vi "Run.vi"(8 "error in (no error)":errorcluster caption="entrée d'erreur (pas d'erreur)", 9 "Y":string[][](array[string]), 10 "X":string[][](array[string]), 11 "Argmin.lvclass":refnum<class "Argmin.lvclass">) -> (0 "error out":errorcluster caption="sortie d'erreur", 2 "Data":T1, 3 "Argmin.lvclass":refnum<class "Argmin.lvclass">)   [LabVIEW 2020, in "Argmin.lvclass"]
doc: "Returns : \n\n- argmin : numpy.ndarray\nY[argmin[i], :] is the row in Y that is closest to X[i, :]."
uses:
  Argmin.lvclass
  Argmin.lvclass/Argmin.ctl
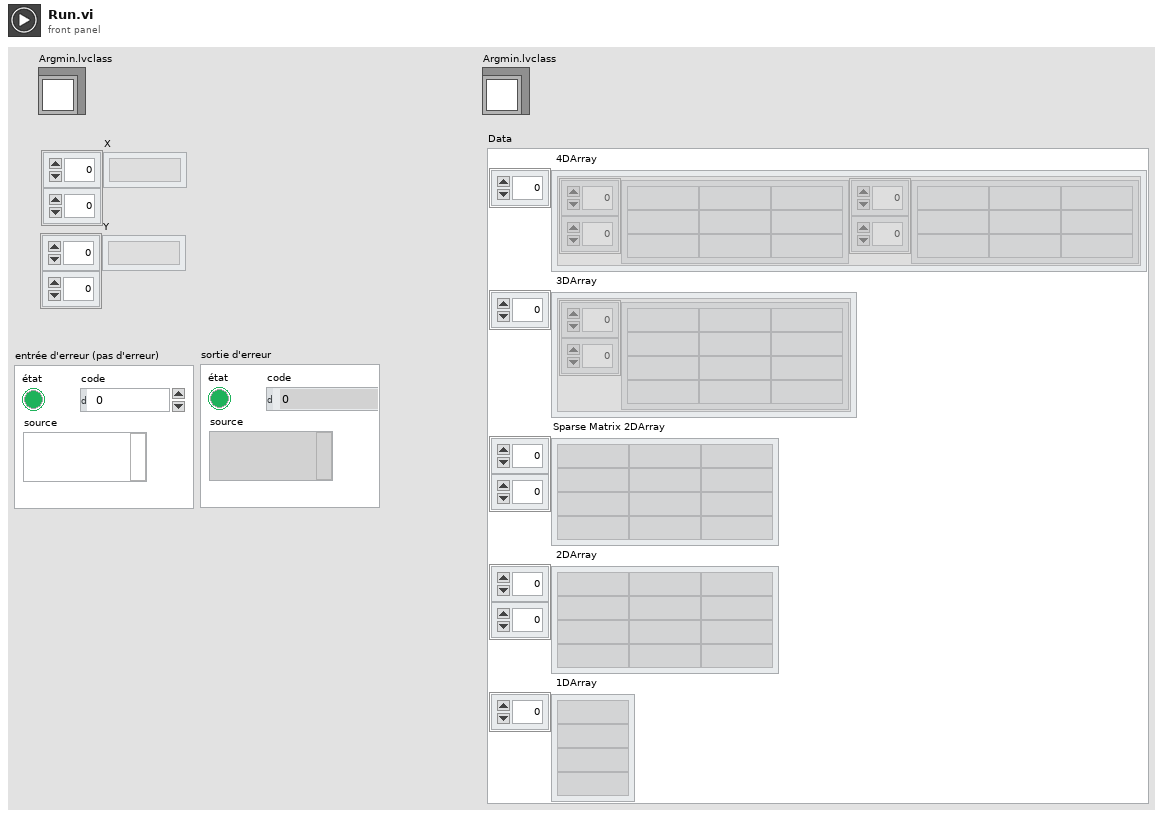
[diagram p1: front panel]
types:
  T1 = cluster{" 4DArray":cluster{"1":string[][], "2":string[][]}[], " 3DArray":cluster{"Tableau":string[][]}[], "Sparse Matrix 2DArray":string[][], " 2DArray":string[][], " 1DArray":string[]}
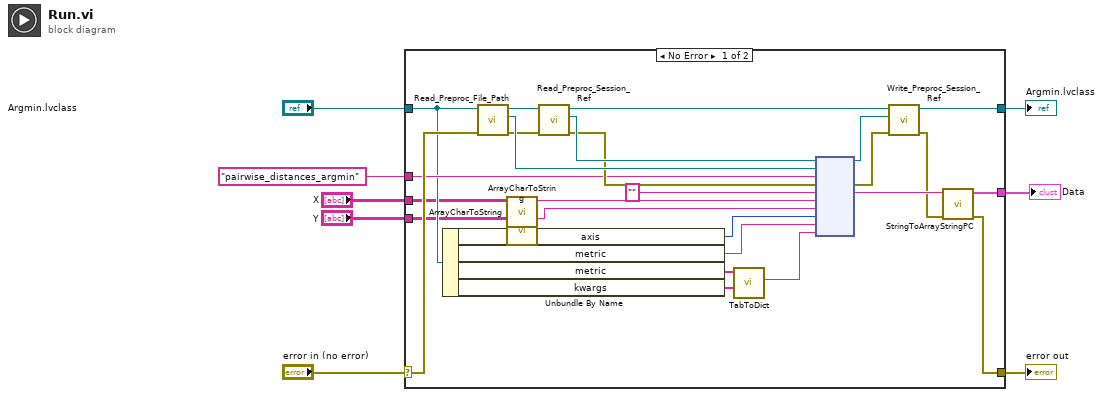
[diagram p0: block diagram]
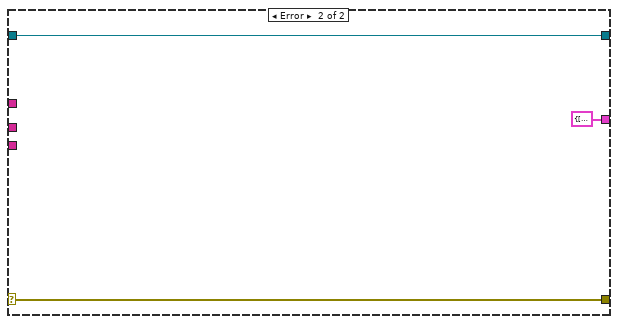
[diagram p2: hidden frame]
diagram:
  n1 = case shown="No Error" "error in (no error)" {
    selector: "error in (no error)" -> [w25 w37]
    tunnel: [w10 w37] -> w7
    tunnel: [w13 w36] -> w5
    tunnel: "Argmin.lvclass" -> [w23 w36]
    tunnel: "pairwise_distances_argmin" ("Fonction") -> [w24 _]
    tunnel: "X" -> [w17 _]
    tunnel: "Y" -> [w16 _]
    tunnel: [w9 T1 {" 4DArray"=[], " 3DArray"=[], "Sparse Matrix 2DArray"=[], " 2DArray"=[], " 1DArray"=[]} ("Data")] -> w1
    frame No Error {
      n2 = Unbundle By Name(w23) -> ("axis"=w22:i32, "metric"=w21:string, "metric"=w20:string[], "kwargs"=w19:string[])
      n3 = call-dynamic "Read_Preproc_File_Path.vi"("error in (no error)"=w25, "Python in"=w23) -> ("error out"=w29:errorcluster, "File_Path"=w32:path, "Python out"=w34:refnum<class "Argmin.lvclass">)  [unwired: 7 in]
      n4 = call "ArrayCharToString.vi"("TAB"=w17) -> ("Instruction"=w15:string)  [unwired: 10 in]
      n5 = call "ArrayCharToString.vi"("TAB"=w16) -> ("Instruction"=w14:string)  [unwired: 10 in]
      n6 = call-dynamic "Read_Preproc_Session_Ref.vi"("error in (no error)"=w29, "Python in"=w34) -> ("error out"=w30:errorcluster, "Session_ref"=w31:refnum<k35>, "Python out"=w33:refnum<class "Argmin.lvclass">)  [unwired: 7 in]
      n7 = call "TabToDict.vi"("String Value"=w19, "String key"=w20) -> ("Dict with string value"=w18:string)  [unwired: 8 in, 1 out]
      n8 = node(w31, w32, w24, w30, "", w15, w14, w22, w21, w18) -> (w26:refnum<k35>, w28:errorcluster, w12:string)  [unwired: 5 in, 2 out]
      n9 = call-dynamic "Write_Preproc_Session_Ref.vi"("error in (no error)"=w28, "Session_ref"=w26, "Python in"=w33) -> ("error out"=w11:errorcluster, "Python out"=w13:refnum<class "Argmin.lvclass">)  [unwired: 7 in]
      n10 = call "StringToArrayStringPC.vi"("sortie d'erreur"=w11, "Return value"=w12) -> ("sortie d'erreur"=w10:errorcluster, "Data"=w9:T1)  [unwired: 8 in]
    }
    frame Error {
    }
  }
  "error out" <- w7
  "Argmin.lvclass" <- w5
  "Data" <- w1
